vi "Configure Blue.vi"(8 "Error In":errorcluster, 11 "eCRDS in":refnum<class "eCRDS.lvclass">) -> (0 "error out":errorcluster, 3 "eCRDS out":refnum<class "eCRDS.lvclass">)   [LabVIEW 2014, in "eCRDS Library.lvlib" / "eCRDS.lvclass"]
doc: "Configure the blue channel for generation and acquisition of the laser signal. The acquisition of the laser signal is run off of a retriggerable clock signal that operates in bursts. When the clock runs, a signal is acquired. The clock only runs when the digital output for the laser goes high. It then generates a finite number of signals until the laser output goes high again.\n\nThe clock for the AI runs off of the same board as the AI. The clock is triggered via a signal run across the backplane on PXI_Trig0 that is connected to the generation signal on the housekeeping card."
uses:
  eCRDS.lvclass
  eCRDS.lvclass/eCRDS.ctl
  reusable/Instrument/Instrument.lvclass/Instrument.ctl
  reusable/Instrument/Read Log Session.vi
  <vilib>/DAQmx/configure/timing.llb/DAQmx Timing (Implicit).vi
  <vilib>/DAQmx/configure/timing.llb/DAQmx Timing (Sample Clock).vi
  <vilib>/DAQmx/configure/trigger.llb/DAQmx Start Trigger (Digital Edge).vi
  <userlib>/_Session Fwk/Session - Root.lvclass
  <resource>/objmgr/daqmx.rc
  reusable/Session APIs/Session Log/System Log.lvclass
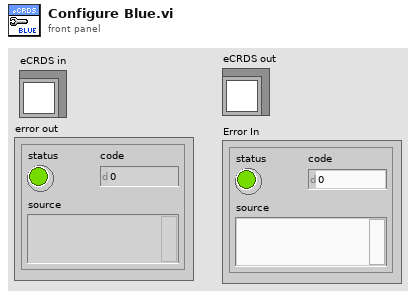
[diagram p1: front panel]
types:
  T1 = typedef "Session - Root.lvclass/Session Handle.ctl" = refnum<data-value>
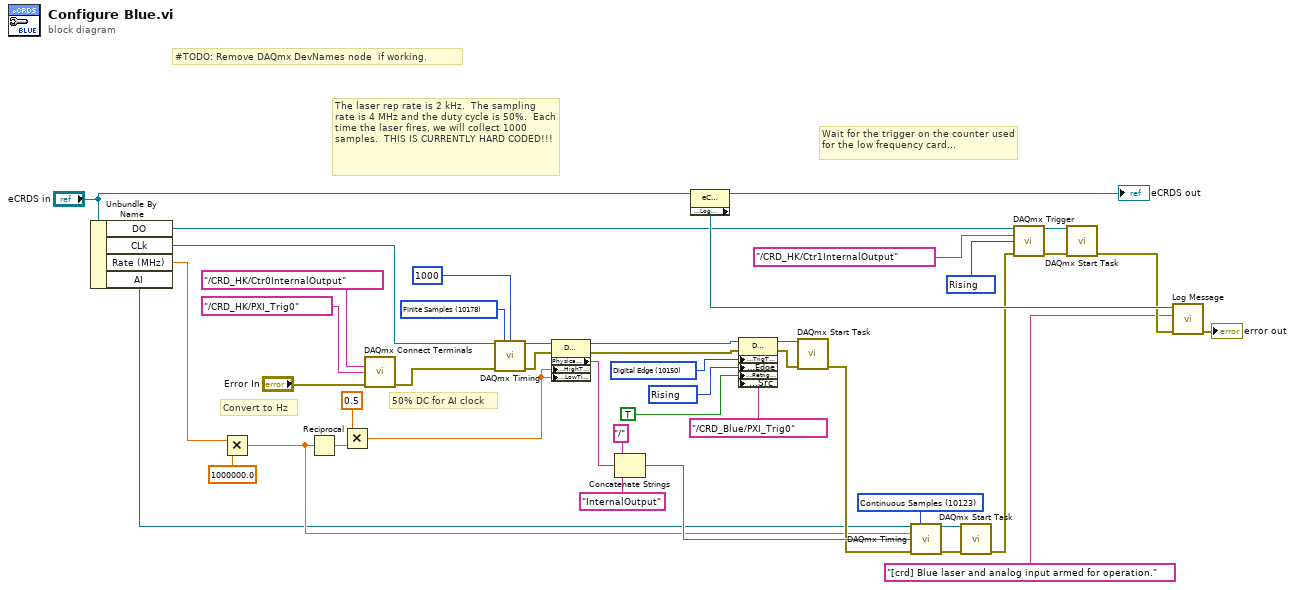
[diagram p0: block diagram]
diagram:
  w1 = 10280 items=["Rising"=10280, "Falling"=10171] ("edge")
  w43 = 10123 items=["Finite Samples"=10178, "Continuous Samples"=10123, "Hardware Timed Single Point"=12522] ("sample mode")
  w34 = 10280 items=["Rising"=10280, "Falling"=10171] ("Ref.DigEdge.Edge")
  w33 = 10150 items=["Analog Edge"=10099, "Digital Edge"=10150, "Digital Pattern"=10398, "Analog Window"=10103, "None"=10230] ("Ref.TrigType")
  w25 = 10178 items=["Finite Samples"=10178, "Continuous Samples"=10123, "Hardware Timed Single Point"=12522] ("sample mode")
  # "The laser rep rate is 2 kHz.  The sampling rate is 4 MHz and the duty cycle is 50%.  Each time the laser fires, we will collect 1000 samples.  THIS IS CURRENTLY HARD CODED!!!"
  # "Wait for the trigger on the counter used for the low frequency card..."
  # "#TODO: Remove DAQmx DevNames node  if working."
  # "50% DC for AI clock"
  # "Convert to Hz"
  n1 = Unbundle By Name("eCRDS in") -> ("DO"=w9:refnum<k21>, "CLk"=w10:refnum<k21>, "Rate (MHz)"=w22:dbl, "AI"=w17:refnum<k21>)
  n2 = Multiply(x=w22, y=1000000.0) -> (x*y=w21:dbl)
  n3 = Reciprocal(x=w21) -> (1/x=w20:dbl)
  n4 = Multiply(x=0.5, y=w20) -> (x*y=w18:dbl)
  n5 = call <vilib>:"DAQmx Connect Terminals.vi"("source terminal"=tag "/CRD_HK/Ctr0InternalOutput", "destination terminal"=tag "/CRD_HK/PXI_Trig0", "error in"="Error In") -> ("error out"=w11:errorcluster)  [unwired: 12 in]
  n6 = call-poly <vilib>:"DAQmx Timing.vi"("task/channels in"=w10, "sample mode"=w25, "samples per channel"=1000, "error in"=w11) -> ("task out"=w27:refnum<k21>, "error out"=w36:errorcluster)  [unwired: 10 in]
  n7 = property class="DAQmx Channel"(reference=w27, error in=w36, "CO.Pulse.HighTime"=w18, "CO.Pulse.LowTime"=w18) -> (reference out=w32:refnum<k21>, error out=w37:errorcluster, "PhysicalChanName"=w30:tag)
  n8 = Concatenate Strings("/" ("string"), w30, "InternalOutput" ("string")) -> (w31:string)
  n9 = property class="eCRDS"(reference="eCRDS in") -> (reference out=→"eCRDS out":refnum<class "eCRDS.lvclass">, "Accessors:Log Session"=w13:T1)  [unwired: 1 in, 1 out]
  n10 = property class="DAQmx Trigger"(reference=w32, error in=w37, "Start.TrigType"=w33, "Start.DigEdge.Edge"=w34, "Start.Retriggerable"=TRUE, "Start.DigEdge.Src"=tag "/CRD_Blue/PXI_Trig0") -> (reference out=w38:refnum<k21>, error out=w39:errorcluster)
  n11 = call <vilib>:"DAQmx Start Task.vi"("task/channels in"=w38, "error in"=w39) -> ("error out"=w24:errorcluster)  [unwired: 12 in, 1 out]
  n12 = call-poly <vilib>:"DAQmx Timing.vi"("task/channels in"=w17, "sample mode"=w43, "rate"=w21, "source"=w31, "error in"=w24) -> ("task out"=w40:refnum<k21>, "error out"=w41:errorcluster)  [unwired: 9 in]
  n13 = call <vilib>:"DAQmx Start Task.vi"("task/channels in"=w40, "error in"=w41) -> ("error out"=w12:errorcluster)  [unwired: 12 in, 1 out]
  n14 = call-poly <vilib>:"DAQmx Trigger.vi"("task/channels in"=w9, "source"=tag "/CRD_HK/Ctr1InternalOutput" ("source terminal"), "edge"=w1, "error in"=w12) -> ("task out"=w44:refnum<k21>, "error out"=w16:errorcluster)  [unwired: 10 in]
  n15 = call <vilib>:"DAQmx Start Task.vi"("task/channels in"=w44, "error in"=w16) -> ("error out"=w5:errorcluster)  [unwired: 12 in, 1 out]
  n16 = call "Log Message.vi"("error in"=w5, "MSG In"="[crd] Blue laser and analog input armed for operation.", "session in"=w13) -> ("error out"=→"error out":errorcluster)  [unwired: 7 in, 1 out]
